vi "Read Response.vi"(8 "error in":errorcluster, 11 "Thorlabs In":refnum<class "Thorlabs.lvclass">) -> (0 "error out":errorcluster, 2 "Success?":bool, 3 "Thorlabs Out":refnum<class "Thorlabs.lvclass">)   [LabVIEW 2018, in "Thorlabs.lvlib" / "Thorlabs.lvclass"]
doc: "This VI Reads the Response from the Device. In this case it just returns True. This is because the error will come through on the Send Command, there is no \"Read Response\" happening in this class.\n\nCreator: Slade Jeppesen\nCreated Date: 09/29/20"
uses:
  Thorlabs.lvclass
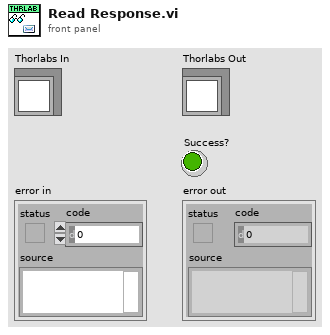
[diagram p1: front panel]
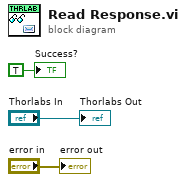
[diagram p0: block diagram]
diagram:
  "error out" <- "error in"
  "Thorlabs Out" <- "Thorlabs In"
  "Success?" <- TRUE ("Success?")
